vi "SSC DCPower Reset Channels.vi"(0 "DCPower SSC in":T1[](array[typedef]), 11 "error in":errorcluster) -> (4 "DCPower SSC out":T1[](array[typedef]), 15 "error out":errorcluster)   [LabVIEW 2020]
doc: "Resets the device to a known state. This VI disables power generation, resets session properties to their default values, commits the session properties, and leaves the sessions in the Uncommitted state. You can use this VI to clear certain errors in less time than using niDCPower Reset Device VI. Refer to the Programming States topic in the NI DC Power Supplies and SMUs Help for more information about NI-DCPower software states."
uses:
  SSC DCPower.ctl
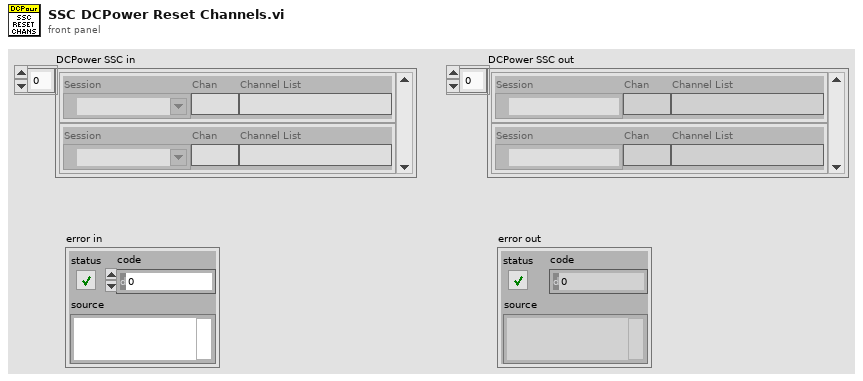
[diagram p1: front panel]
types:
  T1 = typedef "SSC DCPower.ctl" = cluster{"Session":refnum<k15>, "Chan":string, "Channel List":string}
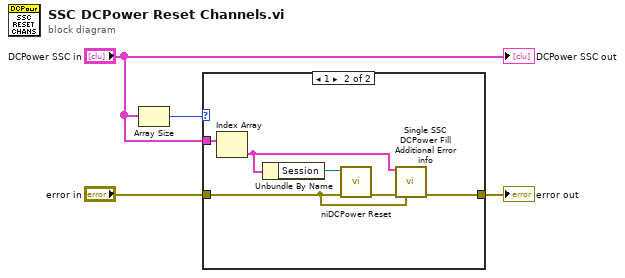
[diagram p0: block diagram]
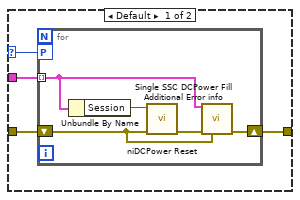
[diagram p2: hidden frame]
diagram:
  n1 = Array Size(array="DCPower SSC in") -> (size(s)=w2:i32)
  n2 = case shown="1" w2 {
    selector: w2 -> [w6 _]
    tunnel: [w8 w19] -> w4
    tunnel: "error in" -> [w7 w18]
    tunnel: "DCPower SSC in" -> [w5 w17]
    frame Default {
      n3 = for {
        tunnel: w5 -> [w10] mode=indexing
        workers-P: w6 -> [_]
        shift-right: [w11] -> w8
        shift-left: w7 -> [w9]
        n4 = Unbundle By Name(w10) -> ("Session"=w12:refnum<k15>)
        n5 = call <instrlib>:"niDCPower Reset.vi"("error in (no error)"=w9, "instrument handle"=w12) -> ("error out"=w13:errorcluster)  [unwired: 8 in, 1 out]
        n6 = call "Single SSC DCPower Fill Additional Error info.vi"("DCPower SSC in"=w10, "error in"=w13, "previous error in"=w9) -> ("error out"=w11:errorcluster)  [unwired: 12 in]
      }
    }
    frame 1 {
      n7 = Index Array(array=w17) -> (element=w14:T1)  [unwired: 1 in]
      n8 = Unbundle By Name(w14) -> ("Session"=w15:refnum<k15>)
      n9 = call <instrlib>:"niDCPower Reset.vi"("error in (no error)"=w18, "instrument handle"=w15) -> ("error out"=w16:errorcluster)  [unwired: 8 in, 1 out]
      n10 = call "Single SSC DCPower Fill Additional Error info.vi"("DCPower SSC in"=w14, "error in"=w16, "previous error in"=w18) -> ("error out"=w19:errorcluster)  [unwired: 12 in]
    }
  }
  "error out" <- w4
  "DCPower SSC out" <- "DCPower SSC in"
